vi "To LabVIEW.vi"(4 "AlbumMap in":refnum<class "AlbumMap.lvclass">, 7 "ExpectedType":refnum<class>, 8 "error in (no error)":errorcluster, 10 "DbRow":variant) -> (0 "error out":errorcluster, 2 "Value":refnum<class>)   [LabVIEW 2020, in "AlbumMap.lvclass"]
uses:
  AlbumMap.lvclass
  C:/Program Files/National Instruments/LabVIEW 2020/vi.lib/Viviota/shared/ORM.lvlibp/ORM/TypeMap/TypeMap.lvclass
  Album/Album.lvclass
  Album/Album.lvclass/Album.ctl
  Album/Write Primary Key.vi
  Album/Write Title.vi
  <vilib>/Viviota/shared/ORM.lvlibp/ORM/TypeMap/Read Autokey.vi
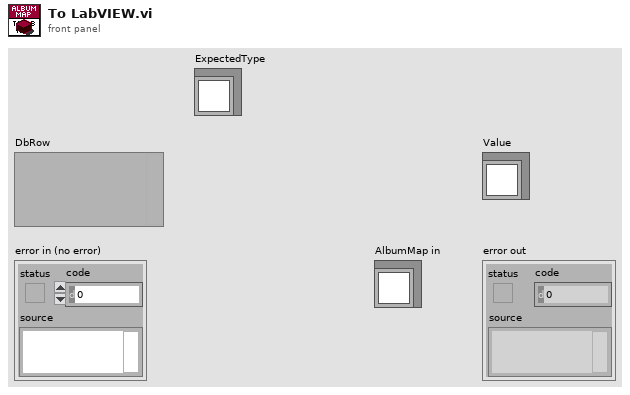
[diagram p1: front panel]
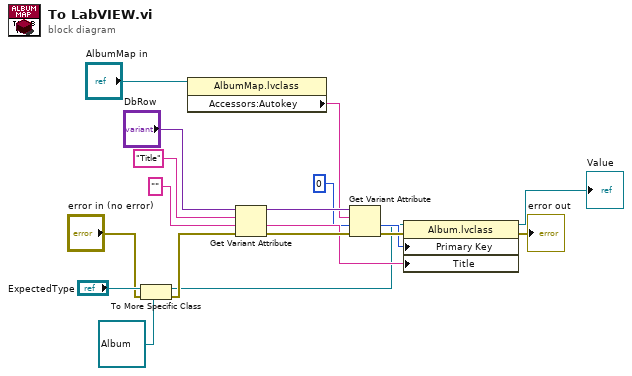
[diagram p0: block diagram]
diagram:
  n1 = To More Specific Class(target class=refnum<class "Album.lvclass"> refnum ("Album.lvclass"), reference="ExpectedType", error in="error in (no error)") -> (specific class reference=w1:refnum<class "Album.lvclass">, error out=w3:errorcluster)
  n2 = property class="AlbumMap.lvclass"(reference="AlbumMap in") -> ("Accessors:Autokey"=w6:string)  [unwired: 1 in, 2 out]
  n3 = Get Variant Attribute(Variant="DbRow", name="Title" ("Title"), default value (empty Variant)="" ("Title"), error in=w3) -> (duplicate Variant=w18:variant, value=w14:string, error out=w16:errorcluster)  [unwired: 1 out]
  n4 = Get Variant Attribute(Variant=w18, name=w6, default value (empty Variant)=i64 0 ("Primary Key"), error in=w16) -> (value=w11:i64, error out=w17:errorcluster)  [unwired: 2 out]
  n5 = property class="Album.lvclass"(reference=w1, error in=w17, "Primary Key"=w11, "Title"=w14) -> (reference out=→"Value":refnum<class "Album.lvclass">, error out=→"error out":errorcluster)
